vi "slscswitch Connect Channels (Single).vi"(8 "error in (no error)":errorcluster, 9 "channel 2":string, 10 "channel 1":string, 11 "SLSC Switch in":refnum<class "SLSC Switch.lvclass">) -> (0 "error out":errorcluster, 3 "SLSC Switch out":refnum<class "SLSC Switch.lvclass">)   [LabVIEW 2015, in "SLSC Switch.lvclass"]
uses:
  SLSC Switch.lvclass
  SLSC Switch.lvclass/SLSC Switch.ctl
  Route Manager/Route Manager.lvclass
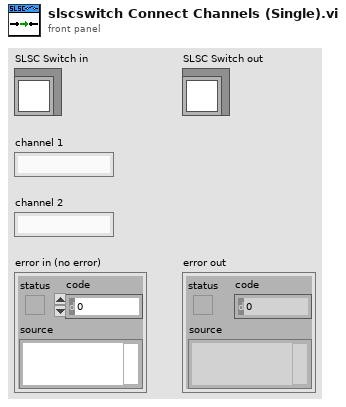
[diagram p1: front panel]
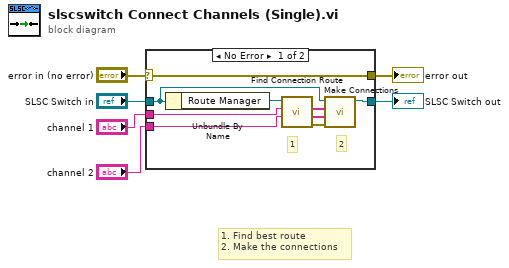
[diagram p0: block diagram]
diagram:
  # "1. Find best route\n2. Make the connections"
  n1 = case shown="No Error" "error in (no error)" {
    selector: "error in (no error)" -> [w15 w17]
    tunnel: [w15 w17] -> w5
    tunnel: [w11 w16] -> w3
    tunnel: "SLSC Switch in" -> [w10 w16]
    tunnel: "channel 1" -> [w8 _]
    tunnel: "channel 2" -> [w7 _]
    frame No Error {
      # "2"
      # "1"
      n2 = Unbundle By Name(w10) -> ("Route Manager"=w9:refnum<class "Route Manager.lvclass">)
      n3 = call "Find Connection Route.vi"("channel 2"=w7, "channel 1"=w8, "Route Manager in"=w9) -> ("error out"=w12:errorcluster, "relays to close"=w13:string[], "relays to open"=w14:string[])  [unwired: 6 in]
      n4 = call "Make Connections.vi"("error in (no error)"=w12, "relays to close"=w13, "relays to open"=w14, "SLSC Switch in"=w10) -> ("SLSC Switch out"=w11:refnum<class "SLSC Switch.lvclass">)  [unwired: 6 in, 1 out]
    }
    frame Error {
    }
  }
  "error out" <- w5
  "SLSC Switch out" <- w3
